vi "SwissSPAD Live_Format SS3 8-bit Gate Pair Data.vi"(8 "Error In":errorcluster, 9 "Y Resolution (250)":i32=250, 11 "Flattened Image (512x256x2)":u8[](array[numeric])) -> (0 "Error Out":errorcluster, 2 "Gate 2 (512x250)":u8[][](array[numeric]), 3 "Integral Gate (512x250)":u8[][](array[numeric]))   [LabVIEW 2021]
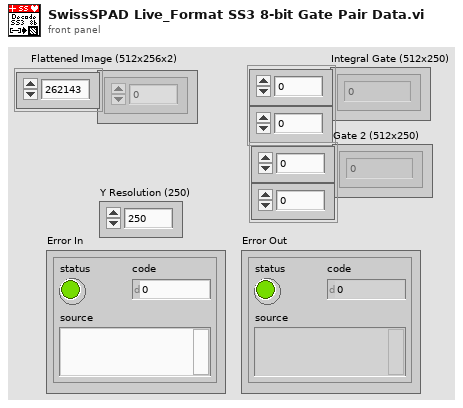
[diagram p1: front panel]
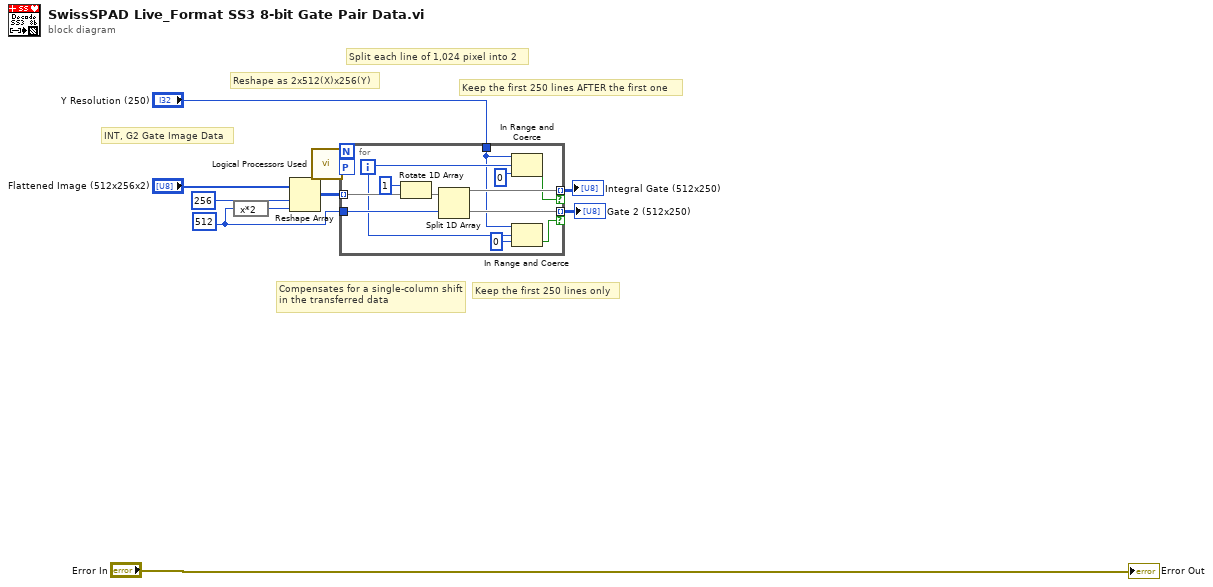
[diagram p0: block diagram]
diagram:
  w1 = 512 ("x")
  # "Compensates for a single-column shift in the transferred data"
  # "Keep the first 250 lines AFTER the first one"
  # "Keep the first 250 lines only"
  # "Split each line of 1,024 pixel into 2"
  # "Reshape as 2x512(X)x256(Y)"
  # "INT, G2 Gate Image Data"
  n1 = expression code="x*2"(w1) -> (w4:i32)
  n2 = Reshape Array("Flattened Image (512x256x2)", 256 ("dimension size"), w4) -> (w8:u8[][])
  n3 = call "Logical Processors Used.vi"() -> ("# Logical Processor Used"=w7:i32)  [unwired: 6 in]
  n4 = for {
    tunnel: w8 -> [w22] mode=indexing
    tunnel: [w21] -> w5 mode=indexing if=w17
    tunnel: [w20] -> w6 mode=indexing if=w14
    workers-P: w7 -> [_]
    tunnel: w1 -> [w19]
    tunnel: "Y Resolution (250)" -> [w13]
    i -> [w16]
    n5 = Rotate 1D Array(1:w22, 2:1 ("n")) -> (0:w12:u8[])
    n6 = Split 1D Array(array=w12, index=w19) -> (first subarray=w21:u8[], second subarray=w20:u8[])
    n7 = In Range and Coerce(upper limit=w13, x=w16, lower limit=0) -> (In Range?=w17:bool)  [unwired: 1 out]
    n8 = In Range and Coerce(upper limit=w13, x=w16, lower limit=0) -> (In Range?=w14:bool)  [unwired: 1 out]
  }
  "Integral Gate (512x250)" <- w5
  "Gate 2 (512x250)" <- w6
  "Error Out" <- "Error In"
